vi "Stop Config.vi"(8 "error in":errorcluster, 11 "PAS in":refnum<class "PAS.lvclass">) -> (0 "error out":errorcluster, 3 "PAS out":refnum<class "PAS.lvclass">)   [LabVIEW 2014, in "PAS.lvclass"]
doc: "Complete the configuration of the PAS. The default does nothing. It is a place holder for tasks such as closing a config file or completing any other processes not covered by the generic methods."
uses:
  PAS.lvclass
  Instrument/state.ctl
  Instrument/Instrument.lvclass
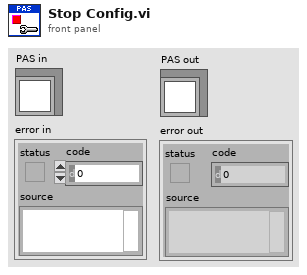
[diagram p1: front panel]
types:
  T1 = typedef "Instrument.lvclass/state.ctl" = enum8{"Configure", "Acquire", "Wait", "Quit", "Handle Error", "NOOP"}
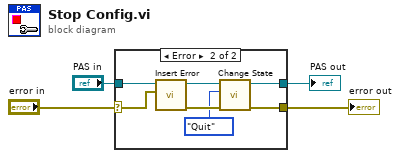
[diagram p0: block diagram]
diagram:
  n1 = case shown="Error" "error in" {
    selector: "error in" -> [w5 w12]
    tunnel: [w5 w7] -> w3
    tunnel: [w6 w8] -> w1
    tunnel: "PAS in" -> [w6 w13]
    frame No Error {
    }
    frame Error {
      n2 = call "Insert Error.vi"("err"=w12, "Instrument in"=w13) -> ("error out"=w10:errorcluster, "Instrument out"=w11:refnum<class "PAS.lvclass">)  [unwired: 7 in, 1 out]
      n3 = call "Change State.vi"("error in"=w10, "instr state"=state."Quit", "Instrument in"=w11) -> ("error out"=w7:errorcluster, "Instrument out"=w8:refnum<class "PAS.lvclass">)  [unwired: 7 in]
    }
  }
  "error out" <- w3
  "PAS out" <- w1
